vi "TEKTRONIK SIGNAL PROCESSING.vi"() -> ()   [LabVIEW 2015]
uses:
  <vilib>/Utility/error.llb/DialogType.ctl
  <instrlib>/Tektronix TDS 200 1000 2000 Series/Public/Data/Read (Single Waveform).vi
  <vilib>/measure/madcrms.llb/Basic Averaged DC-RMS for 1 Chan.vi
  <vilib>/express/express analysis/Spectral/Block/exnSpectralBlock spectral measurements peak poly.vi
  <vilib>/express/express analysis/Spectral/Block/exnSpectralBlock spectral measurements peak WFM.vi
  <vilib>/express/express analysis/Spectral/XNode/ExpressSpectralMeasurementsBlockNode.xnode
  <instrlib>/Tektronix TDS 200 1000 2000 Series/Tektronix TDS 200 1000 2000 Series.lvlib
  <vilib>/measure/NI_MAPro.lvlib
panel:
  out "DATE TIME":string
  out "TIME":string
  in  "OPERATOR":string
  in  "JUDUL":string
  in  "SPEED (S)":i32
  in  "SAVE DATA":bool
  in  "FILE FOLDER":path
  in  "Tab Control":enum32{"Page 1", "Page 2"}(tab)
  out "WG":waveform(dbl)(graph)
  out "FFT":cluster{"f0":dbl, "df":dbl, "magnitude":dbl[]}(graph)
  out "Cluster":T1
  out "Data array":dbl[](array[numeric])
  in  "VISA resource name":refnum<visa-resource-name>
  in  "Reset":bool
  # "SIGNAL PROCESSING USING TEXTRONIK DIGITAL OCILOSCOPE TDS 1000 SERRIES"
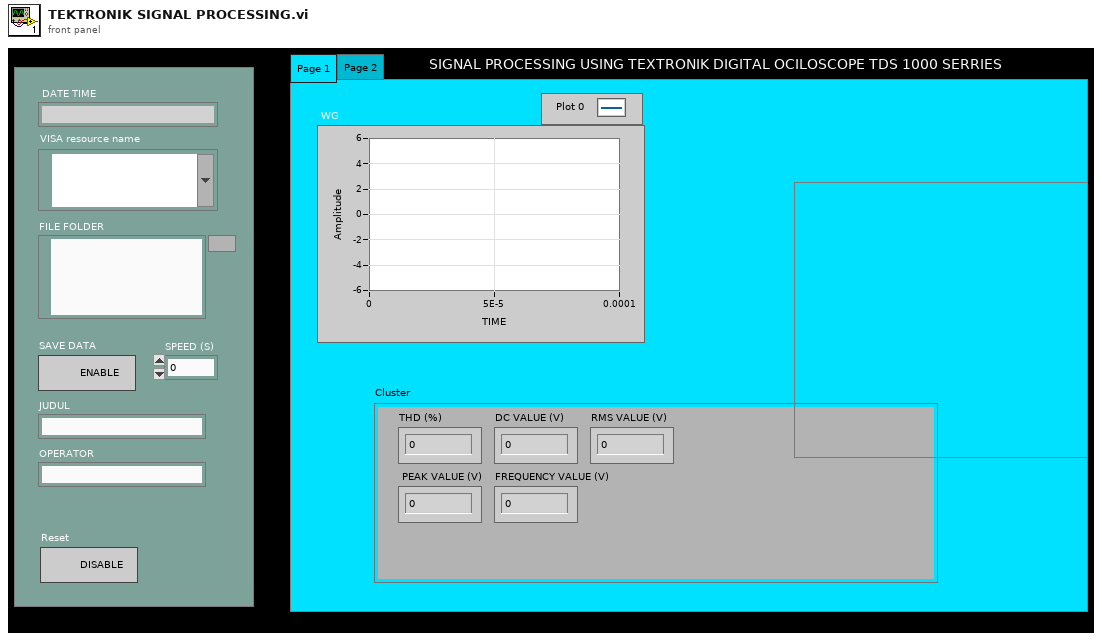
[diagram p1: front panel]
types:
  T1 = cluster{"THD (%)":dbl, "DC VALUE (V)":dbl, "RMS VALUE (V) ":dbl, " PEAK VALUE (V)":dbl, "FREQUENCY VALUE (V) ":dbl}
  T2 = enum16{"open", "replace", "create", "open or create", "replace or create", "replace or create with confirmation"}
  T3 = typedef "DialogType.ctl" = u16
  T4 = cluster{"Baud Rate":u32, "Parity":u16, "Stop Bits":u16, "Flow Control":u16}
  T5 = enum16{"Rectangular (none)", "Hanning", "Low side lobe"}
  T6 = cluster{"averaging mode":u16, "weighting mode":u16, "number of averages":u32}
  T7 = cluster{"dB On (F)":bool, "unwrap phase (F)":bool, "convert to degree (F)":bool}
  T8 = cluster{dbl, "DC value":dbl, "RMS value":dbl, "Scalar":dbl, "Scalar":dbl}
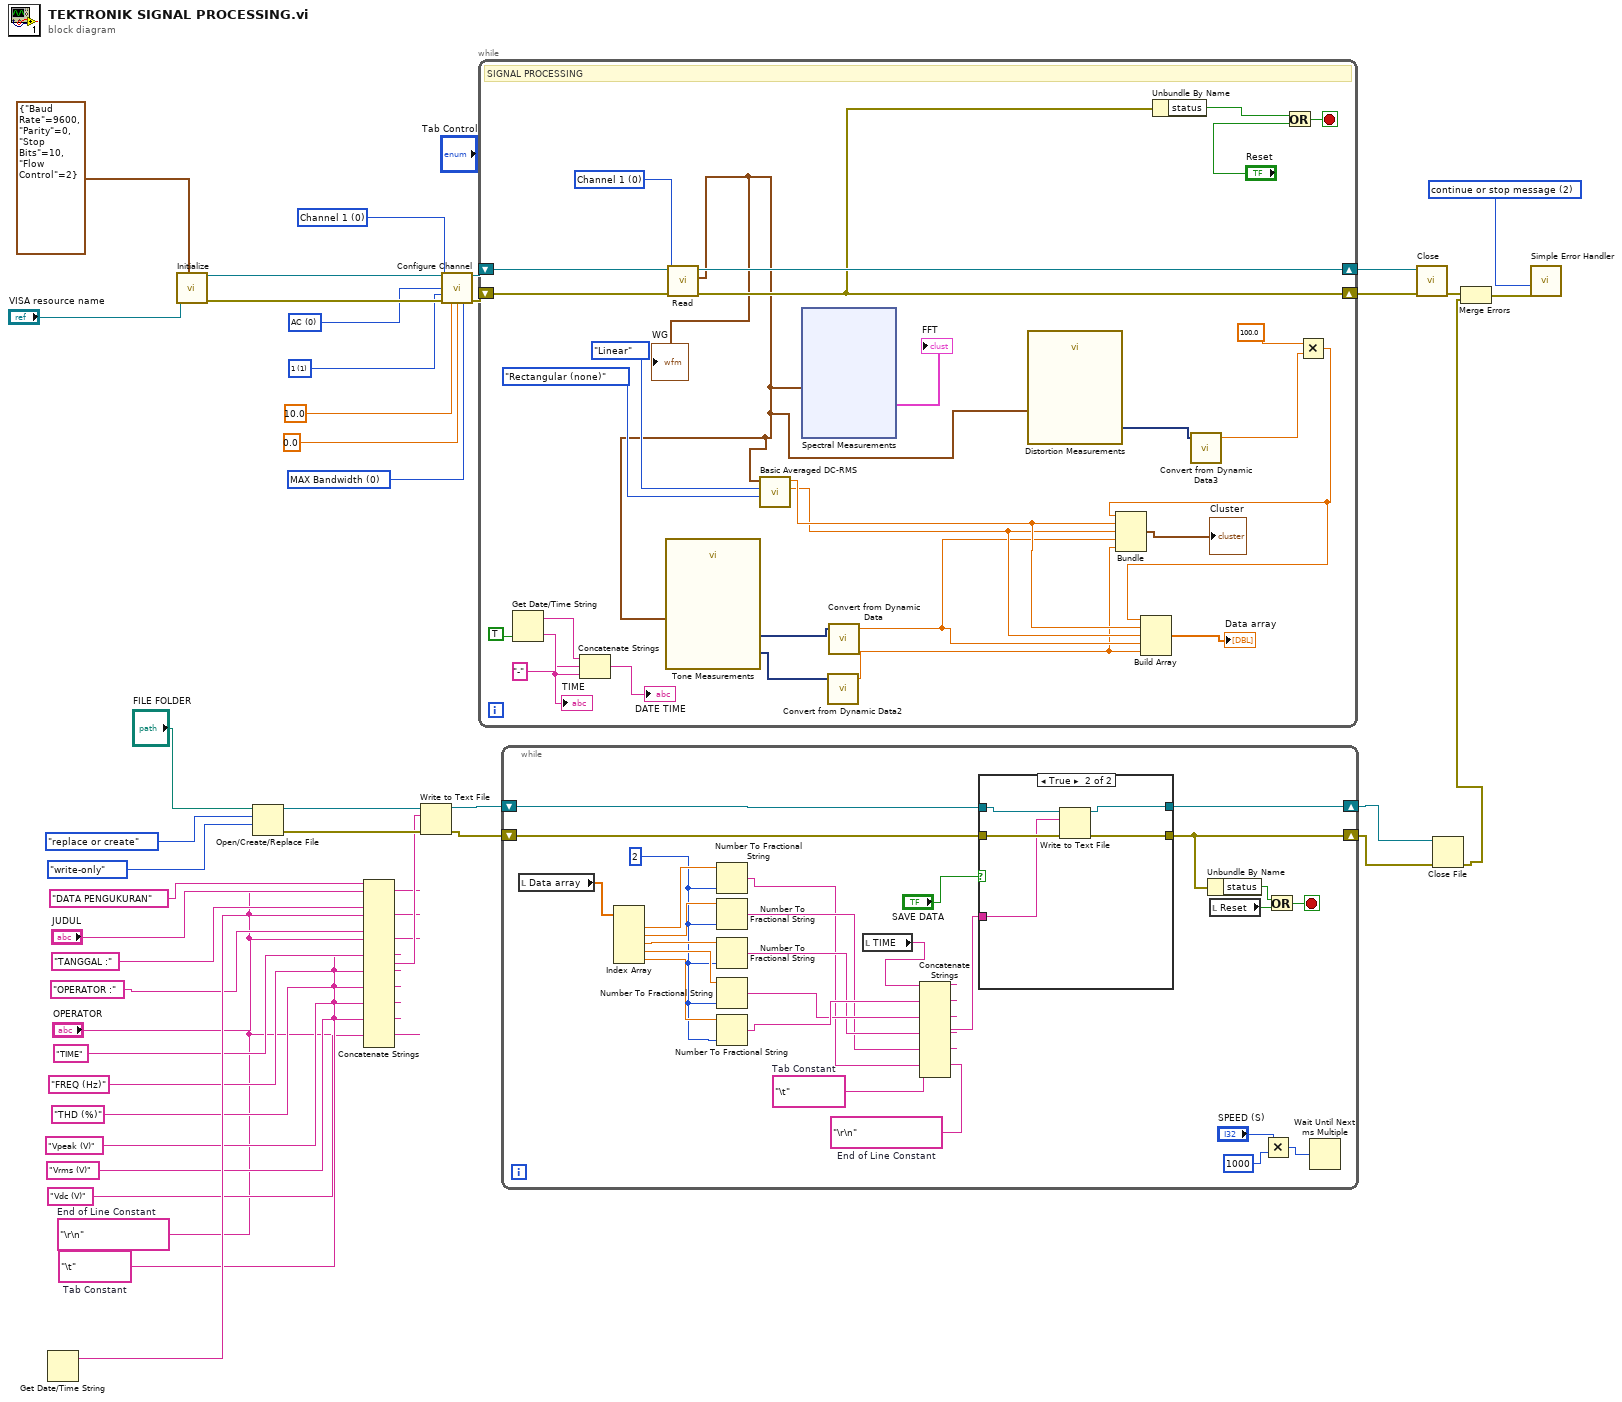
[diagram p0: block diagram]
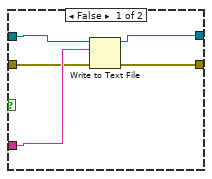
[diagram p2: hidden frame]
diagram:
  w3 = "\t"  # Tab Constant
  w1 = "\r\n"  # End of Line Constant
  w29 = T3 2 items=["no dialog", "OK message", "continue or stop message", "OK message + warnings", "continue/stop + warnings"] ("type of dialog (OK msg:1)")
  w35 = 0 items=["Channel 1", "Channel 2", "Channel 3", "Channel 4", "Math", "Reference A", "Reference B", "Reference C", "Reference D"] ("Channel (0: Channel 1)")
  w36 = 0 items=["AC", "DC", "Ground"] ("Vertical Coupling (1: DC)")
  w37 = 1 items=["1"=1, "10"=10, "20"=20, "50"=50, "100"=100, "500"=500, "1000"=1000] ("Probe Attenuation (10: 10X)")
  w39 = 0 items=["MAX Bandwidth", "Unlimited"] ("Bandwidth (0: MAX Bandwidth)")
  n1 = Get Date/Time String() -> (date string=w11:string)  [unwired: 3 in, 1 out]
  n2 = call <instrlib>:"Initialize.vi"("Serial Configuration"=T4 {"Baud Rate"=9600, "Parity"=0, "Stop Bits"=10, "Flow Control"=2}, "VISA resource name"="VISA resource name") -> ("error out"=w38:errorcluster, "VISA resource name out"=w34:refnum<visa-resource-name>)  [unwired: 8 in]
  n3 = Open/Create/Replace File(file path (use dialog)="FILE FOLDER", operation (0:open)=T2."replace or create", access (0:read/write)=enum16{"read/write", "read-only", "write-only"}."write-only") -> (refnum out=w24:refnum<file>, error out=w23:errorcluster)  [unwired: 3 in, 1 out]
  n4 = Concatenate Strings "Concatenate Strings"("DATA PENGUKURAN" ("string"), "JUDUL", w1, "TANGGAL :" ("string"), w11, w1, "OPERATOR :" ("string"), "OPERATOR", w1, "TIME" ("string"), w3, "FREQ (Hz)" ("string"), w3, "THD (%)" ("string"), w3, "Vpeak (V)" ("string"), w3, "Vrms (V)" ("string"), w3, "Vdc (V)" ("string"), w1) -> (w15:string)
  n5 = Write to Text File(file (use dialog)=w24, text=w15, error in=w23) -> (refnum out=w26:refnum<file>, error out=w25:errorcluster)  [unwired: 1 in, 1 out]
  n6 = call <instrlib>:"Configure Channel.vi"("VISA resource name"=w34, "Channel (0: Channel 1)"=w35, "Vertical Coupling (1: DC)"=w36, "Probe Attenuation (10: 10X)"=w37, "error in (no error)"=w38, "Vertical Range (10.0 V/div)"=10.0, "Vertical Offset (0.0 divs)"=0.0, "Bandwidth (0: MAX Bandwidth)"=w39) -> ("VISA resource name out"=w33:refnum<visa-resource-name>, "error out"=w32:errorcluster)  [unwired: 6 in]
  n7 = while {
    shift-right: [w69] -> w31
    shift-left: w33 -> [w71]
    shift-right: [w64] -> w30
    shift-left: w32 -> [w70]
    stop <- w68 stop-if-true
    w58 = u16 0 items=["Channel 1", "Channel 2", "Channel 3", "Channel 4", "Math", "Reference A", "Reference B", "Reference C", "Reference D", "FFT"] ("Source (0: Channel 1)")
    # "SIGNAL PROCESSING"
    n8 = Get Date/Time String(want seconds? (F)=TRUE) -> (date string=w47:string, time string=w45:string)  [unwired: 2 in]
    "TIME" <- w45
    n9 = Concatenate Strings(w47, "-" ("string"), w45) -> (→"DATE TIME":string)
    n10 = call-poly <instrlib>:"Read.vi"("error in (no error)"=w70, "Source (0: Channel 1)"=w58, "VISA resource name"=w71) -> ("error out"=w64:errorcluster, "Waveform Data"=w48:waveform(dbl), "VISA resource name out"=w69:refnum<visa-resource-name>)  [unwired: 6 in]
    "WG" <- w48
    n11 = call "Tone Measurements"("Signals"=w48) -> ("Frequency"=w62:dynamicdata, "Amplitude"=w63:dynamicdata)  [unwired: 8 in, 1 out]
    n12 = call-poly <vilib>:"Basic Averaged DC-RMS.vi"("window"=T5."Rectangular (none)", "averaging type"=enum16{"Linear", "Exponential"}."Linear", "signal in"=w48) -> ("RMS value"=w53:dbl, "DC value"=w54:dbl)  [unwired: 5 in, 2 out]
    n13 = xnode "Spectral Measurements"("Signals"=w48) -> ("FFT - (Peak)"=→"FFT":cluster{"f0":dbl, "df":dbl, "magnitude":dbl[]})  [unwired: 1 in, 2 out]
    n14 = call "Convert from Dynamic Data2"("Dynamic Data Type"=w62) -> ("Scalar"=w49:dbl)  [unwired: 3 in]
    n15 = call "Convert from Dynamic Data"("Dynamic Data Type"=w63) -> ("Scalar"=w50:dbl)  [unwired: 3 in]
    n16 = call "Distortion Measurements"("Signals"=w48) -> ("THD"=w59:dynamicdata)  [unwired: 9 in, 1 out]
    n17 = Unbundle By Name "Unbundle By Name"(w64) -> ("status"=w67:bool)
    n18 = call "Convert from Dynamic Data3"("Dynamic Data Type"=w59) -> ("Scalar"=w57:dbl)  [unwired: 3 in]
    n19 = Or(x=w67, y="Reset") -> (x .or. y?=w68:bool)
    n20 = Multiply(x=100.0, y=w57) -> (x*y=w55:dbl)
    n21 = Bundle "Bundle"(w55, "DC value"=w54, "RMS value"=w53, "Scalar"=w50, "Scalar"=w49) -> (→"Cluster":T8)  [unwired: 1 in]
    n22 = Build Array "Build Array"(w55, w54, w53, w50, w49) -> (→"Data array":dbl[])
  }
  n23 = while {
    shift-right: [w83] -> w19
    shift-left: w26 -> [w108]
    shift-right: [w82] -> w20
    shift-left: w25 -> [w107]
    stop <- w106 stop-if-true
    w85 = "\r\n"  # End of Line Constant
    w87 = "\t"  # Tab Constant
    w93 = 2
    n24 = local read "Data array"() -> (w92:dbl[])
    n25 = Index Array "Index Array"(array=w92) -> (element #1=w105:dbl, element #2=w104:dbl, element #3=w103:dbl, element #4=w102:dbl, element #5=w101:dbl)  [unwired: 5 in]
    n26 = Number To Fractional String(number=w105, precision (6)=w93) -> (F-format string=w86:string)  [unwired: 2 in]
    n27 = Number To Fractional String(number=w104, precision (6)=w93) -> (F-format string=w88:string)  [unwired: 2 in]
    n28 = Number To Fractional String(number=w103, precision (6)=w93) -> (F-format string=w89:string)  [unwired: 2 in]
    n29 = Number To Fractional String(number=w102, precision (6)=w93) -> (F-format string=w90:string)  [unwired: 2 in]
    n30 = Number To Fractional String(number=w101, precision (6)=w93) -> (F-format string=w91:string)  [unwired: 2 in]
    n31 = local read "TIME"() -> (w84:string)
    n32 = Concatenate Strings(w84, w87, w91, w87, w90, w87, w89, w87, w88, w87, w86, w85) -> (w94:string)
    n33 = case shown="True" "SAVE DATA" {
      tunnel: w108 -> [w113 w118]
      tunnel: w107 -> [w111 w117]
      tunnel: w94 -> [w112 w116]
      tunnel: [w110 w114] -> w83
      tunnel: [w109 w115] -> w82
      frame False {
        n34 = Write to Text File(file (use dialog)=w113, text=w112, error in=w111) -> (refnum out=w110:refnum<file>, error out=w109:errorcluster)  [unwired: 1 in, 1 out]
      }
      frame True {
        n35 = Write to Text File(file (use dialog)=w118, text=w116, error in=w117) -> (refnum out=w114:refnum<file>, error out=w115:errorcluster)  [unwired: 1 in, 1 out]
      }
    }
    n36 = Unbundle By Name(w82) -> ("status"=w99:bool)
    n37 = local read "Reset"() -> (w95:bool)
    n38 = Multiply(x="SPEED (S)", y=1000) -> (x*y=w98:i32)
    n39 = Or(x=w99, y=w95) -> (x .or. y?=w106:bool)
    n40 = Wait Until Next ms Multiple(millisecond multiple=w98) -> ()  [unwired: 1 out]
  }
  n41 = call <instrlib>:"Close.vi"("error in (no error)"=w30, "VISA resource name"=w31) -> ("error out"=w18:errorcluster)  [unwired: 9 in]
  n42 = Close File(refnum=w19, error in=w20) -> (error out=w16:errorcluster)  [unwired: 1 out]
  n43 = Merge Errors(w18, w16) -> (w17:errorcluster)
  n44 = call <vilib>:"Simple Error Handler.vi"("type of dialog (OK msg:1)"=w29, "error in (no error)"=w17) -> ()  [unwired: 3 in, 5 out]
